vi "Update Device List.vi"(8 "error in":errorcluster, 10 "Device Table Strings":string[][](array[string]), 11 "VF Device Selection in":refnum<class "VF Device Selection.lvclass">) -> (0 "error out":errorcluster, 3 "VF Device Selection out":refnum<class "VF Device Selection.lvclass">)   [LabVIEW 2018, in "VF Device Selection Actor.lvlib" / "VF Device Selection.lvclass"]
uses:
  VF Device Selection.lvclass
  VF Device Selection.lvclass/VF Device Selection.ctl
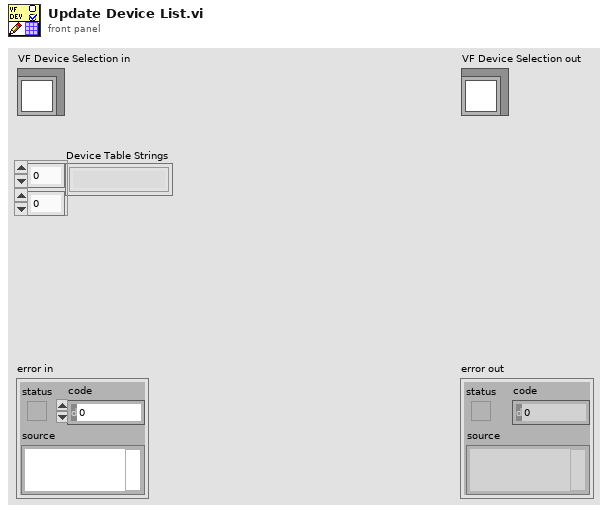
[diagram p1: front panel]
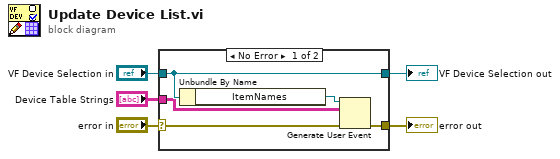
[diagram p0: block diagram]
diagram:
  n1 = case shown="No Error" "error in" {
    selector: "error in" -> [w7 w12]
    tunnel: [w8 w12] -> w4
    tunnel: [w10 w11] -> w2
    tunnel: "VF Device Selection in" -> [w10 w11]
    tunnel: "Device Table Strings" -> [w6 _]
    frame No Error {
      n2 = Unbundle By Name(w10) -> ("ItemNames"=w9:refnum<user-event>)
      n3 = Generate User Event(user event=w9, event data cluster=w6, error in=w7) -> (error out=w8:errorcluster)  [unwired: 1 in, 1 out]
    }
    frame Error {
    }
  }
  "error out" <- w4
  "VF Device Selection out" <- w2
